vi "SHA-1.vi"(8 "error in (no error)":errorcluster, 11 "Message":string="The quick brown fox jumps over the lazy dog") -> (0 "error out":errorcluster, 1 "ASCII Formatted hash":string, 3 "binary string hash":string)   [LabVIEW 2012, in "Encryption.lvlib"]
uses:
  Encryption.lvlib
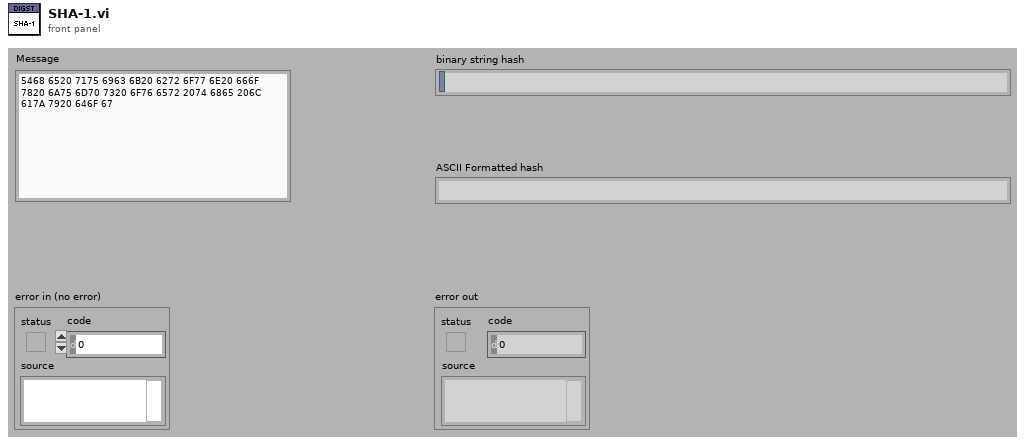
[diagram p1: front panel]
types:
  T1 = enum16{"big-endian, network order", "native, host order", "little-endian"}
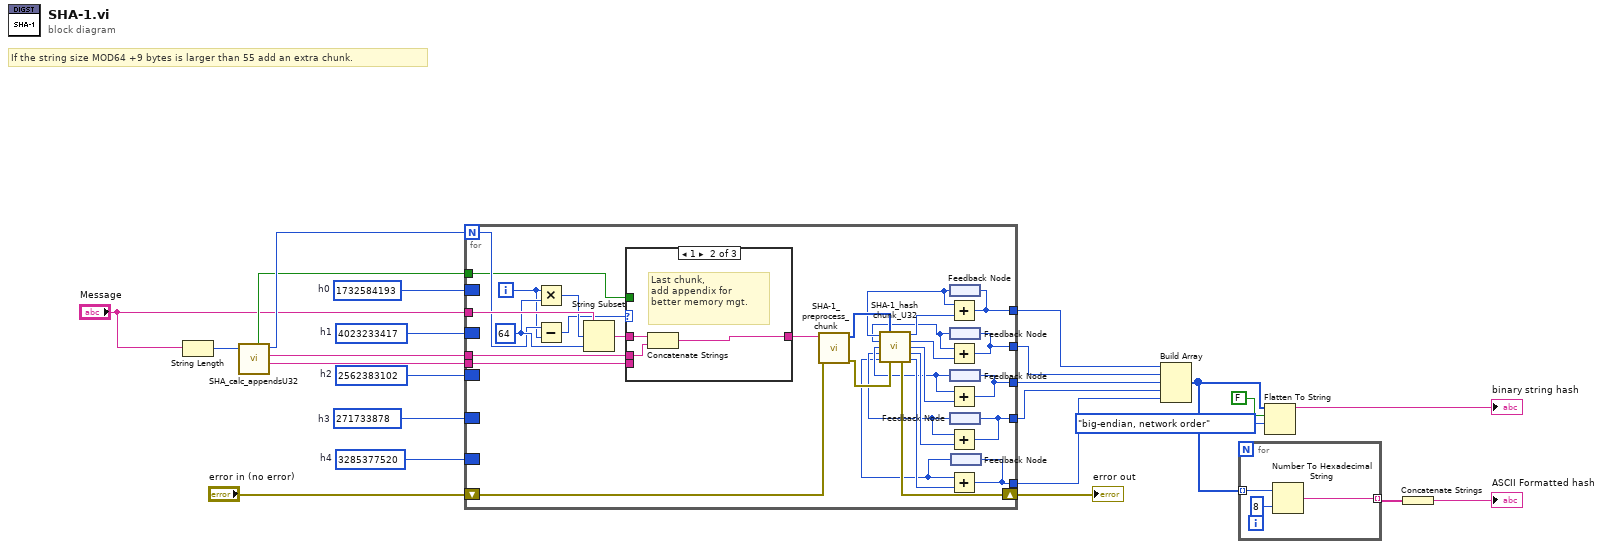
[diagram p0: block diagram]
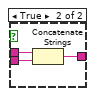
[diagram p4: hidden frame]
diagram:
  w12 = u32 3285377520  # h4
  w13 = u32 271733878  # h3
  w14 = u32 2562383102  # h2
  w15 = u32 4023233417  # h1
  w16 = u32 1732584193  # h0
  # "If the string size MOD64 +9 bytes is larger than 55 add an extra chunk."
  n1 = String Length(string="Message") -> (length=w8:i32)
  n2 = call "SHA_calc_appendsU32.vi"("String length"=w8) -> ("Second last chunk"=w9:string, "Last Chunk"=w1:string, "Number of chunks"=w11:i32, "Double appends"=w10:bool)  [unwired: 7 in]
  n3 = for {
    N: w11 -> [w51]
    tunnel: "Message" -> [w54]
    tunnel: w1 -> [w47]
    tunnel: [w45] -> w24
    tunnel: [w44] -> w23
    tunnel: [w43] -> w22
    tunnel: [w42] -> w21
    tunnel: [w46] -> w20
    border: w12 -> [_]
    border: w16 -> [_]
    border: w15 -> [_]
    border: w14 -> [_]
    border: w13 -> [_]
    tunnel: w10 -> [w36]
    tunnel: w9 -> [w35]
    shift-right: [w34] -> w7
    shift-left: "error in (no error)" -> [w33]
    i -> [w50]
    w52 = 64 ("x")
    n4 = Multiply(x=w50, y=w52) -> (x*y=w53:i32)
    n5 = Subtract(x=w51, y=w50) -> (x-y=w48:i32)
    n6 = String Subset(string=w54, offset (0)=w53, length (rest)=w52) -> (substring=w49:string)
    n7 = case shown="1" w48 {
      tunnel: w49 -> [w55 w58 w62]
      tunnel: [w55 w56 w61] -> w25
      tunnel: w47 -> [_ w57 _]
      tunnel: w35 -> [_ _ w60]
      tunnel: w36 -> [_ _ w59]
      frame Default {
        # "Not last chunk"
      }
      frame 1 {
        # "Last chunk,\nadd appendix for\nbetter memory mgt."
        n8 = Concatenate Strings(w58, w57) -> (w56:string)
      }
      frame 2 {
        # "Second last chunk,\nmight need appendix"
        n9 = case shown="假" w59 {
          tunnel: w62 -> [w63 w66]
          tunnel: [w63 w65] -> w61
          tunnel: w60 -> [_ w64]
          frame False {
          }
          frame True {
            n10 = Concatenate Strings(w66, w64) -> (w65:string)
          }
        }
      }
    }
    n11 = call "SHA-1_preprocess_chunk.vi"("error in (no error)"=w33, "Chunk in"=w25) -> ("error out"=w31:errorcluster, "Processed chunk out"=w32:u32[])  [unwired: 8 in]
    n12 = feedback #1() -> (w30:u32)
    n13 = feedback #2() -> (w29:u32)
    n14 = feedback #3() -> (w28:u32)
    n15 = feedback #4() -> (w27:u32)
    n16 = feedback #5() -> (w26:u32)
    n17 = call "SHA-1_hash chunk_U32.vi"("h0"=w30, "Chunk"=w32, "h1"=w29, "h2"=w28, "h3"=w27, "h4"=w26, "error in (no error)"=w31) -> ("a"=w41:u32, "b"=w40:u32, "c"=w39:u32, "d"=w38:u32, "error out"=w34:errorcluster, "e"=w37:u32)  [unwired: 3 in]
    n18 = Add(x=w30, y=w41) -> (x+y=w45:u32)
    n19 = Add(x=w29, y=w40) -> (x+y=w44:u32)
    n20 = Add(x=w28, y=w39) -> (x+y=w43:u32)
    n21 = Add(x=w27, y=w38) -> (x+y=w42:u32)
    n22 = Add(x=w26, y=w37) -> (x+y=w46:u32)
    n23 = feedback-in #1(w45) -> ()
    n24 = feedback-in #2(w44) -> ()
    n25 = feedback-in #3(w43) -> ()
    n26 = feedback-in #4(w42) -> ()
    n27 = feedback-in #5(w46) -> ()
  }
  "error out" <- w7
  n28 = Build Array(w24, w23, w22, w21, w20) -> (w5:u32[])
  n29 = for {
    tunnel: w5 -> [w69] mode=indexing
    tunnel: [w67] -> w4 mode=indexing
    n30 = Number To Hexadecimal String(1:i16 8 ("width (-)"), 2:w69) -> (0:w67:string)
  }
  n31 = Flatten To String(anything=w5, prepend array or string size? (T)=FALSE, byte order (0:big-endian, network order)=T1."big-endian, network order") -> (data string=→"binary string hash":string)  [unwired: 1 in, 2 out]
  n32 = Concatenate Strings(w4) -> (→"ASCII Formatted hash":string)
